vi "Teleop.vi"(9 "Match Info":T1={"Autonomous Elapsed Seconds"=0.0, "TeleOp Elapsed Seconds"=0.0, "Disabled Elapsed Seconds"=0.0, "Visited Autonomous"=FALSE, "Visited TeleOp"=FALSE, "Visited Disabled"=FALSE, "Autonomous Settings"={"Autonomous Style"=enum."Independent", "VI Refnum"=refnum}}, 11 "Call Context":T2) -> (0 "LeftOutput":dbl, 3 "RightOutput":dbl)   [LabVIEW 2014]
doc: "This VI is called for each TeleOp packet received from the DS where the robot is not disabled. It is often used to read from the joysticks and update I/O or to update setpoints for timed control loops. It should complete and return within 20 milliseconds or it may miss DS packets."
uses:
  <vilib>/Rock Robotics/WPI/DriverStation/WPI_DriverStationDerivedRobotMode.ctl
  <vilib>/Rock Robotics/WPI/DriverStation/WPI_DriverStationMatch Info.ctl
  Robot Global Data.vi
  <vilib>/Rock Robotics/WPI/RobotDrive/WPI_RobotDriveGetSetRefNum.vi
  <vilib>/addons/control/pid/pid.llb/PID Control Input Filter (DBL).vi
  <vilib>/addons/control/pid/pid.llb/PID (DBL).vi
  <vilib>/addons/control/pid/NI_PID_pid.lvlib
panel:
  out "error out":errorcluster
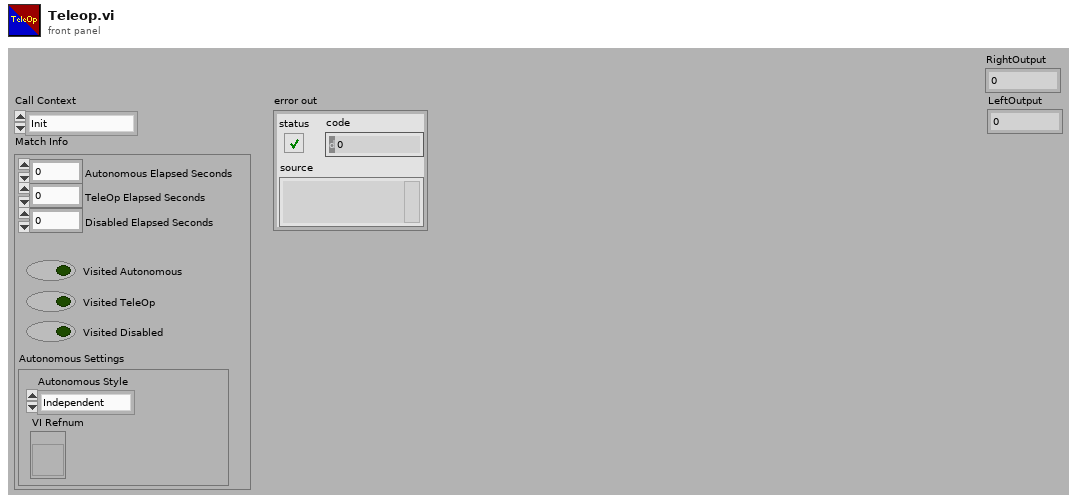
[diagram p1: front panel]
types:
  T1 = typedef "WPI_DriverStationMatch Info.ctl" = cluster{"Autonomous Elapsed Seconds":dbl, "TeleOp Elapsed Seconds":dbl, "Disabled Elapsed Seconds":dbl, "Visited Autonomous":bool, "Visited TeleOp":bool, "Visited Disabled":bool, "Autonomous Settings":cluster{"Autonomous Style":enum16{"Iterative", "Independent"}, "VI Refnum":refnum<vi>}}
  T2 = typedef "WPI_DriverStationDerivedRobotMode.ctl" = enum16{"Init", "Execute", "Stop"}
  T3 = typedef "WPI_RobotDriveDevRef.ctl" = cluster{"DevStatus":errorcluster, "Motors[]":T4[], "Square Inputs":bool, "Max Output":dbl}
  T4 = typedef "WPI_MotorControlDeviceRef.ctl" = cluster{"DeviceStatus":errorcluster, "Type":enum16{"PWM", "CAN"}, "PWM":cluster{"Controller":T5, "PWM Channel":T6, "DeadBand":T7}, "CAN":cluster{"Device Number":u8, "Control Mode":T8, "Semaphore":T9, "Max Vout":dbl}, "Invert":bool, "TransformRef":T10, "InvTransformRef":T10}
  T5 = typedef "FPGA_TypedefDigitalModule.ctl" = enum16{"Controller 1"}
  T6 = typedef "FPGA_DIOPWMChannel.ctl" = enum8{"PWM 0", "PWM 1", "PWM 2", "PWM 3", "PWM 4", "PWM 5", "PWM 6", "PWM 7", "PWM 8", "PWM 9", "PWM MXP 0", "PWM MXP 1", "PWM MXP 2", "PWM MXP 3", "PWM MXP 4", "PWM MXP 5", "PWM MXP 6", "PWM MXP 7", "PWM MXP 8", "PWM MXP 9", "Invalid"}
  T7 = typedef "WPI_PWMDeadband.ctl" = cluster{"Name":string, "maxPositivePwm":i32, "minPositivePwm":i32, "centerPwm":i32, "maxNegativePwm":i32, "minNegativePwm":i32, "angularRange":u16}
  T8 = typedef "WPI_CANJaguar_ControlMode.ctl" = enum8{"Percent VBus", "Current", "Speed", "Position", "Voltage"}
  T9 = typedef "Semaphore RefNum" = refnum<k1>
  T10 = typedef "WPI_PWMTransform_ConPane.ctl" = refnum<vi>
  T11 = typedef "WPI_GyroDevRef.ctl" = cluster{"DevStatus":errorcluster, "Analog Module":T12, "Analog Channel":T13, "Offset":dbl, "Gain (VoltsPerDegree/Second)":dbl}
  T12 = typedef "FPGA_TypedefAnalogModule.ctl" = enum16{"Controller 1"}
  T13 = typedef "FPGA_AIChannel.ctl" = enum8{"AI 0", "AI 1", "AI 2", "AI 3", "AI MXP 0", "AI MXP 1", "AI MXP 2", "AI MXP 3", "Invalid"}
  T14 = cluster{"X":bool, "A":bool, "B":bool, "Y":bool, "LB":bool, "RB":bool, "LT":bool, "RT":bool, "Back":bool, "Start":bool, "LC":bool, "RC":bool}
  T15 = cluster{"Up":bool, "Down":bool, "Left":bool, "Right":bool}
  T16 = cluster{"proportional gain (Kc)":dbl, "integral time (Ti, min)":dbl, "derivative time (Td, min)":dbl}
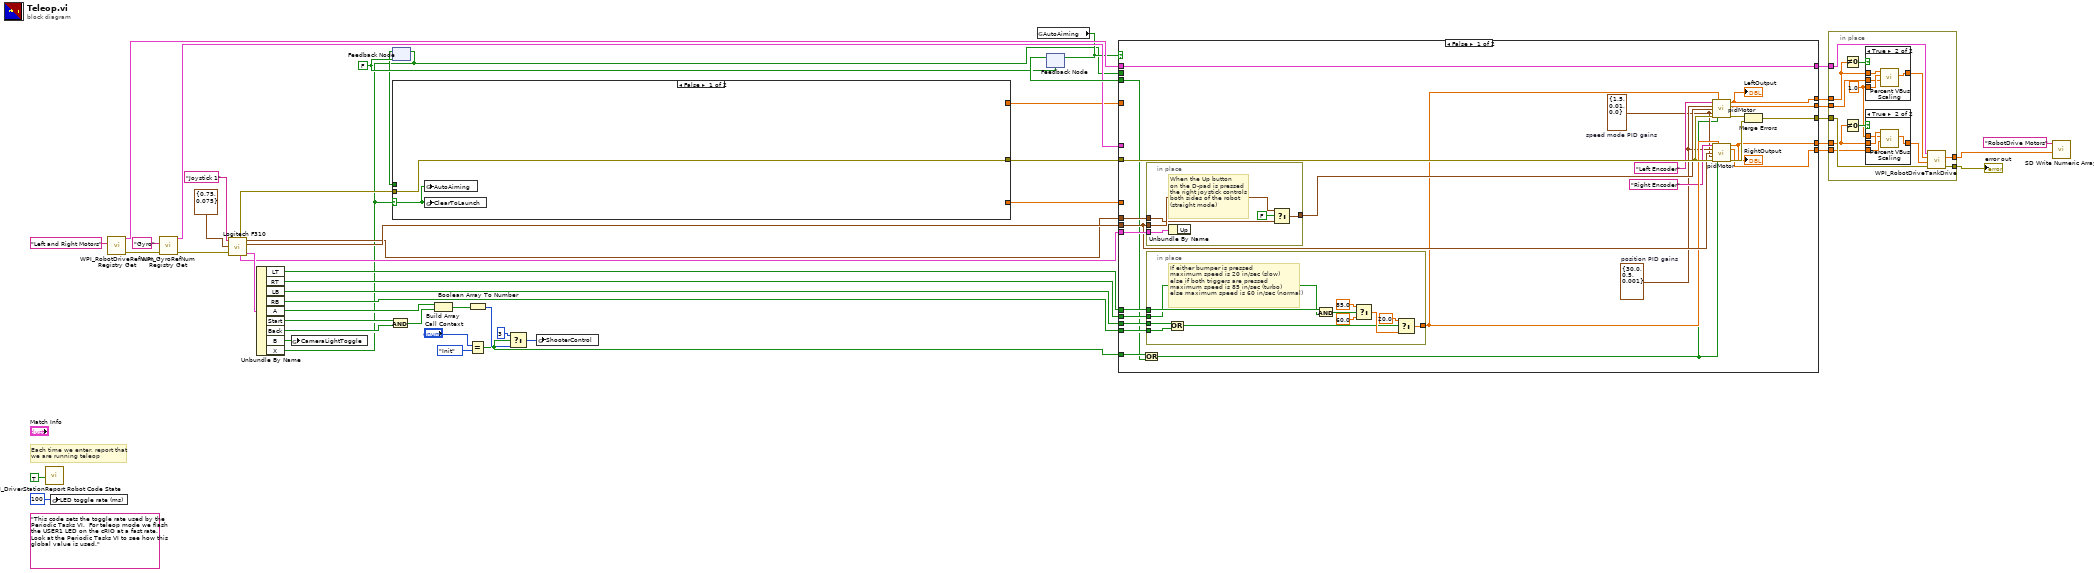
[diagram p0: block diagram]
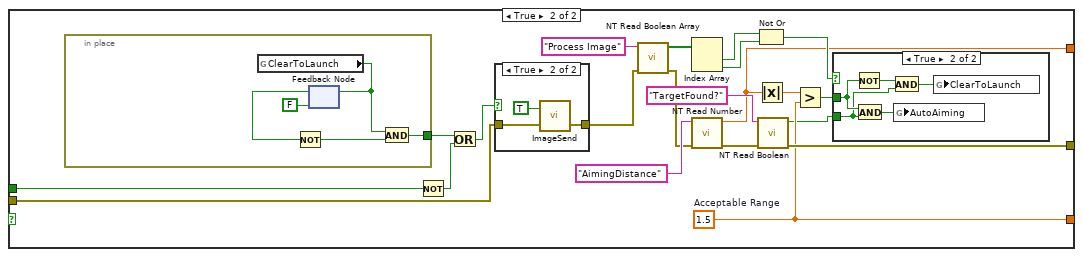
[diagram p4: hidden frame]
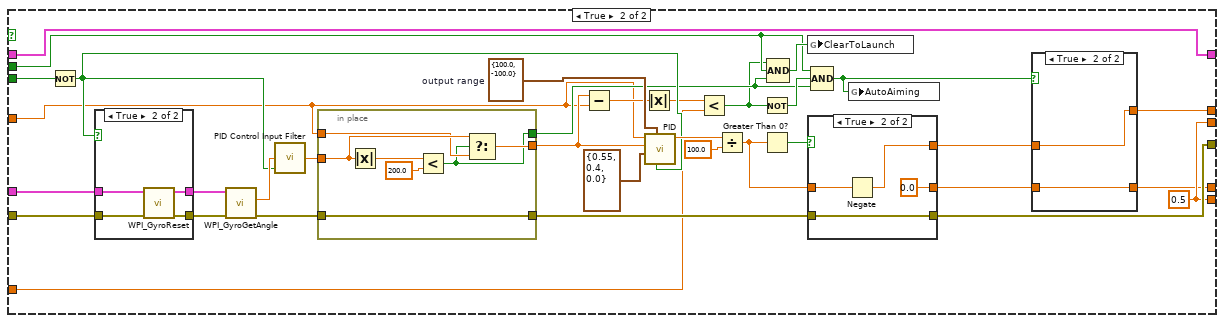
[diagram p7: hidden frame]
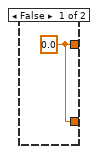
[diagram p8: hidden frame]
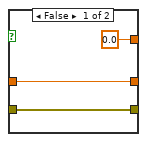
[diagram p10: hidden frame]
diagram:
  w12 = FALSE ("X")
  (unwired) "This code sets the toggle rate used by the Periodic Tasks VI.  For teleop mode we flash the USER1 LED on the cRIO at a fast rate.  Look at the Periodic Tasks VI to see how this global value is used."
  # "Each time we enter, report that\nwe are running teleop"
  n1 = call <vilib>:"WPI_DriverStationReport Robot Code State.vi"("TeleOp"=TRUE ("Autonomous")) -> ()  [unwired: 10 in, 1 out]
  n2 = global write "Robot Global Data.vi" "LED toggle rate (ms)"(u32 100 ("LED ms toggle rate")) -> ()
  n3 = call <vilib>:"WPI_RobotDriveRefNum Registry Get.vi"("refnum name"="Left and Right Motors") -> ("error out"=w29:errorcluster, "RobotDriveDevRef"=w30:T3)  [unwired: 9 in]
  n4 = call <vilib>:"WPI_GyroRefNum Registry Get.vi"("error in (no error)"=w29, "refnum name"="Gyro") -> ("error out"=w13:errorcluster, "GyroDevRef"=w14:T11)  [unwired: 8 in]
  n5 = call "Logitech F310.vi"("error in (no error)"=w13, "Deadzone Scale Cluster"=cluster{"Scale":dbl, "Deadzone":dbl} {"Scale"=0.75, "Deadzone"=0.075}, "refnum name"="Joystick 1") -> ("Buttons"=w43:T14, "D-Pad Buttons"=w15:T15, "Right Stick"=w32:cluster{"X":dbl, "Y":dbl}, "error out"=w10:errorcluster, "Left Stick"=w31:cluster{"X":dbl, "Y":dbl})  [unwired: 1 in]
  n6 = Unbundle By Name(w43) -> ("LT"=w42:bool, "RT"=w41:bool, "LB"=w40:bool, "RB"=w39:bool, "A"=w28:bool, "Start"=w36:bool, "Back"=w35:bool, "B"=w24:bool, "X"=w5:bool)
  n7 = global write "Robot Global Data.vi" "CameraLightToggle"(w24) -> ()
  n8 = And(x=w36, y=w35) -> (x .and. y?=w37:bool)
  n9 = feedback-in #1(w5) -> ()
  n10 = feedback #1(w12) -> (w11:bool)
  n11 = case shown="False" w5 {
    selector: w5 -> [w49 _]
    tunnel: w11 -> [_ w71]
    tunnel: w10 -> [w50 w70]
    tunnel: [w50 w68] -> w9
    tunnel: [_ w51] -> w8
    tunnel: [_ w63] -> w4
    frame False {
      n12 = global write "Robot Global Data.vi" "AutoAiming"(w49) -> ()
      n13 = global write "Robot Global Data.vi" "ClearToLaunch"(w49) -> ()
    }
    frame True {
      w63 = 1.5  # Acceptable Range
      n14 = in-place {
        in-place-border: [w72] -> w61
        n15 = global read "Robot Global Data.vi" "ClearToLaunch"() -> (w74:bool)
        n16 = feedback-in #2(w74) -> ()
        n17 = feedback #2(FALSE ("ClearToLaunch")) -> (w73:bool)
        n18 = Not(x=w73) -> (.not. x?=w75:bool)
        n19 = And(x=w74, y=w75) -> (x .and. y?=w72:bool)
      }
      n20 = Not(x=w71) -> (.not. x?=w60:bool)
      n21 = Or(x=w61, y=w60) -> (x .or. y?=w67:bool)
      n22 = case shown="True" w67 {
        tunnel: w70 -> [w82 w83]
        tunnel: [w82 w85] -> w69
        frame False {
        }
        frame True {
          n23 = call "ImageSend.vi"("error in (no error)"=w83, "mode (T=AutoAim, F=HotGoal)"=TRUE) -> ("error out"=w85:errorcluster)  [unwired: 1 in]
        }
      }
      n24 = call <vilib>:"NT Read Boolean Array.vi"("error in"=w69, "Name"="Process Image") -> ("error out"=w58:errorcluster, "Boolean Array"=w56:bool[])  [unwired: 8 in]
      n25 = Index Array(array=w56) -> (element #1=w55:bool, element #2=w54:bool)  [unwired: 2 in]
      n26 = call <vilib>:"NT Read Number.vi"("error in"=w58, "Name"="AimingDistance") -> ("error out"=w52:errorcluster, "Numeric"=w51:dbl)  [unwired: 8 in]
      n27 = Not Or(1:w54, 2:w55) -> (0:w53:bool)
      n28 = Absolute Value(x=w51) -> (abs(x)=w64:dbl)
      n29 = call <vilib>:"NT Read Boolean.vi"("error in"=w52, "Name"="TargetFound?") -> ("error out"=w68:errorcluster, "Boolean"=w59:bool)  [unwired: 8 in]
      n30 = Greater?(x=w64, y=w63) -> (0:w62:bool)
      n31 = case shown="True" w53 {
        tunnel: w62 -> [_ w80]
        tunnel: w59 -> [_ w78]
        frame False {
        }
        frame True {
          n32 = Not(x=w80) -> (.not. x?=w77:bool)
          n33 = And(x=w80, y=w78) -> (x .and. y?=w81:bool)
          n34 = And(x=w77, y=w78) -> (x .and. y?=w79:bool)
          n35 = global write "Robot Global Data.vi" "AutoAiming"(w81) -> ()
          n36 = global write "Robot Global Data.vi" "ClearToLaunch"(w79) -> ()
        }
      }
    }
  }
  n37 = Build Array(w28, w37) -> (w38:bool[])
  n38 = Equal?(x="Call Context", y=WPI_DriverStationDerivedRobotMode."Init") -> (x = y?=w23:bool)
  n39 = Boolean Array To Number(Boolean array=w38) -> (number=w27:u32)
  n40 = Select(t=u32 3, s=w23, f=w27) -> (s? t:f=w26:u32)
  n41 = global write "Robot Global Data.vi" "ShooterControl"(w26) -> ()
  n42 = global read "Robot Global Data.vi" "AutoAiming"() -> (w7:bool)
  n43 = feedback-in #3(w7) -> ()
  n44 = feedback #3(w12) -> (w22:bool)
  n45 = case shown="False" w7 {
    tunnel: w9 -> [w110 w148]
    tunnel: w42 -> [w109 _]
    tunnel: w41 -> [w108 _]
    tunnel: w40 -> [w107 _]
    tunnel: w39 -> [w106 _]
    tunnel: w15 -> [w105 _]
    tunnel: w32 -> [w103 _]
    tunnel: w31 -> [w102 _]
    tunnel: w30 -> [w90 w152]
    tunnel: w23 -> [w94 _]
    tunnel: w22 -> [w92 w155]
    tunnel: w14 -> [_ w149]
    tunnel: [w91 w153] -> w20
    tunnel: [w87 w138] -> w17
    tunnel: [w86 w139] -> w18
    tunnel: [w90 w152] -> w19
    tunnel: [w89 w144] -> w16
    tunnel: w8 -> [_ w128]
    tunnel: [w88 w144] -> w6
    tunnel: w5 -> [_ w142]
    tunnel: w4 -> [_ w130]
    frame False {
      w95 = T16 {"proportional gain (Kc)"=1.5, "integral time (Ti, min)"=0.01, "derivative time (Td, min)"=0.0}  # speed mode PID gains
      w96 = T16 {"proportional gain (Kc)"=30.0, "integral time (Ti, min)"=0.5, "derivative time (Td, min)"=0.001}  # position PID gains
      n46 = Or(x=w94, y=w92) -> (x .or. y?=w93:bool)
      n47 = in-place {
        in-place-border: w105 -> [w126]
        in-place-border: [w125] -> w104
        in-place-border: w103 -> [w124]
        in-place-border: w102 -> [w123]
        # "When the Up button\non the D-pad is pressed\nthe right joystick controls\nboth sides of the robot \n(straight mode)"
        n48 = Unbundle By Name(w126) -> ()  [unwired: 1 out]
        n49 = Select(t=w124, s=FALSE, f=w123) -> (s? t:f=w125:cluster{"X":dbl, "Y":dbl})
      }
      n50 = in-place {
        in-place-border: [w121] -> w99
        in-place-border: w109 -> [w120]
        in-place-border: w108 -> [w119]
        in-place-border: w107 -> [w114]
        in-place-border: w106 -> [w113]
        # "If either bumper is pressed\nmaximum speed is 20 in/sec (slow)\nelse if both triggers are pressed\nmaximum speed is 85 in/sec (turbo)\nelse maximum speed is 60 in/sec (normal)"
        n51 = Or(x=w114, y=w113) -> (x .or. y?=w112:bool)
        n52 = And(x=w120, y=w119) -> (x .and. y?=w118:bool)
        n53 = Select(t=85.0, s=w118, f=60.0 ("x")) -> (s? t:f=w117:dbl)
        n54 = Select(t=20.0 ("Multiplier"), s=w112, f=w117) -> (s? t:f=w121:dbl)
      }
      n55 = call "pidMotor.vi"("Encoder"="Left Encoder" ("refnum name"), "Multiplier"=w99, "position PID gains"=w96, "Joystic  cluster"=w104, "speed mode PID gains"=w95, "error in (no error)"=w110, "Init?"=w93) -> ("output"=w86:dbl, "minimum % vbus"=w89:dbl, "error out"=w100:errorcluster)  [unwired: 4 in, 2 out]
      "LeftOutput" <- w86
      n56 = call "pidMotor.vi"("Encoder"="Right Encoder" ("refnum name"), "Multiplier"=w99, "position PID gains"=w96, "Joystic  cluster"=w103, "speed mode PID gains"=w95, "error in (no error)"=w110, "Init?"=w93) -> ("output"=w87:dbl, "minimum % vbus"=w88:dbl, "error out"=w101:errorcluster)  [unwired: 4 in, 2 out]
      "RightOutput" <- w87
      n57 = Merge Errors(w100, w101) -> (w91:errorcluster)
    }
    frame True {
      w144 = 0.5 ("Numeric")
      w157 = cluster{"output high":dbl, "output low":dbl} {"output high"=100.0, "output low"=-100.0}  # output range
      n58 = Not(x=w155) -> (.not. x?=w146:bool)
      n59 = case shown="True" w146 {
        tunnel: [w172 w176] -> w150
        tunnel: w149 -> [w172 w173]
        tunnel: w148 -> [w171 w175]
        tunnel: [w171 w174] -> w147
        frame False {
        }
        frame True {
          n60 = call <vilib>:"WPI_GyroReset.vi"("error in (no error)"=w175, "GyroDevRef"=w173) -> ("error out"=w174:errorcluster, "GyroDevRef"=w176:T11)  [unwired: 8 in]
        }
      }
      n61 = call <vilib>:"WPI_GyroGetAngle.vi"("error in (no error)"=w147, "GyroDevRef"=w150) -> ("error out"=w134:errorcluster, "Angle"=w156:dbl)  [unwired: 6 in, 2 out]
      n62 = call-poly <vilib>:"PID Control Input Filter.vi"("reinitialize? (F)"=w146, "input"=w156) -> ("output"=w127:dbl)  [unwired: 3 in]
      n63 = in-place {
        in-place-border: w127 -> [w165]
        in-place-border: [w164] -> w133
        in-place-border: [w162] -> w136
        in-place-border: w128 -> [w163]
        in-place-border: [w161] -> w135
        in-place-border: w134 -> [w161]
        n64 = Absolute Value(x=w165) -> (abs(x)=w167:dbl)
        n65 = Less?(x=w167, y=200.0) -> (x < y?=w162:bool)
        n66 = Select(t=w165, s=w162, f=w163) -> (s? t:f=w164:dbl)
      }
      n67 = Subtract(x=w133, y=w128) -> (x-y=w132:dbl)
      n68 = Absolute Value(x=w132) -> (abs(x)=w131:dbl)
      n69 = call-poly <vilib>:"PID.vi"("reinitialize? (F)"=w146, "output range"=w157, "PID gains"=T16 {"proportional gain (Kc)"=0.55, "integral time (Ti, min)"=0.4, "derivative time (Td, min)"=0.0}, "process variable"=w133, "setpoint"=w128) -> ("output"=w159:dbl)  [unwired: 5 in, 1 out]
      n70 = Less?(x=w131, y=w130) -> (x < y?=w129:bool)
      n71 = Divide(x=w159, y=100.0) -> (x/y=w151:dbl)
      n72 = Not(x=w129) -> (.not. x?=w145:bool)
      n73 = Greater Than 0?(x=w151) -> (x > 0?=w154:bool)
      n74 = Compound Arithmetic op=AND(w129, w142, w136) -> (w143:bool)
      n75 = global write "Robot Global Data.vi" "ClearToLaunch"(w143) -> ()
      n76 = case shown="True" w154 {
        tunnel: w135 -> [w179 w182]
        tunnel: [w179 w182] -> w153
        tunnel: w151 -> [w177 w183]
        tunnel: [w177 0.0] -> w137
        tunnel: [0.0 ("-x") w180] -> w140
        frame False {
        }
        frame True {
          n77 = Negate(x=w183) -> (-x=w180:dbl)
        }
      }
      n78 = Compound Arithmetic op=AND(w142, w145, w136) -> (w141:bool)
      n79 = global write "Robot Global Data.vi" "AutoAiming"(w141) -> ()
      n80 = case shown="True" w141 {
        tunnel: w140 -> [_ w170]
        tunnel: [w168 w170] -> w139
        tunnel: [w168 w169] -> w138
        tunnel: w137 -> [_ w169]
        frame False {
          w168 = 0.0 ("-x")
        }
        frame True {
        }
      }
    }
  }
  n81 = in-place {
    in-place-border: w20 -> [w196]
    in-place-border: w19 -> [w195]
    in-place-border: w18 -> [w194]
    in-place-border: w17 -> [w191]
    in-place-border: w16 -> [w187]
    in-place-border: w6 -> [w186]
    in-place-border: [w185] -> w3
    in-place-border: [w184] -> w2
    w188 = 1.0 ("Max Percent VBus")
    n82 = Not Equal To 0?(x=w194) -> (x != 0?=w193:bool)
    n83 = Not Equal To 0?(x=w191) -> (x != 0?=w190:bool)
    n84 = case shown="True" w193 {
      tunnel: w194 -> [w202 w206]
      tunnel: [w202 w204] -> w192
      tunnel: w188 -> [_ w205]
      tunnel: w187 -> [_ w203]
      frame False {
      }
      frame True {
        n85 = call "Percent VBus Scaling.vi"("Min %VBus"=w203, "Max %VBus"=w205, "input (1 to -1)"=w206) -> ("output"=w204:dbl)  [unwired: 8 in]
      }
    }
    n86 = case shown="True" w190 {
      tunnel: w191 -> [w197 w201]
      tunnel: [w197 w199] -> w189
      tunnel: w188 -> [_ w200]
      tunnel: w186 -> [_ w198]
      frame False {
      }
      frame True {
        n87 = call "Percent VBus Scaling.vi"("Min %VBus"=w198, "Max %VBus"=w200, "input (1 to -1)"=w201) -> ("output"=w199:dbl)  [unwired: 8 in]
      }
    }
    n88 = call <vilib>:"WPI_RobotDriveTankDrive.vi"("error in (no error)"=w196, "Right axis value"=w189, "Left axis value"=w192, "RobotDriveDevRef"=w195) -> ("error out"=w185:errorcluster, "Motor Values"=w184:dbl[])  [unwired: 5 in, 1 out]
  }
  "error out" <- w3
  n89 = call <vilib>:"SD Write Numeric Array.vi"("Numeric Array"=w2, "Name"="RobotDrive Motors") -> ()  [unwired: 8 in, 2 out]
